vi "DataProcessScaleAdjust.vi"(8 "error in (no error)":errorcluster, 10 "Graph":dbl[](array[numeric]), 11 "Graph":refnum<vi>) -> (0 "error out":errorcluster, 3 "reference out":refnum<vi>)   [LabVIEW 2013, in "main.lvlib"]
uses:
  main.lvlib
  <vilib>/Utility/miscctls.llb/LVRangeTypeDef.ctl
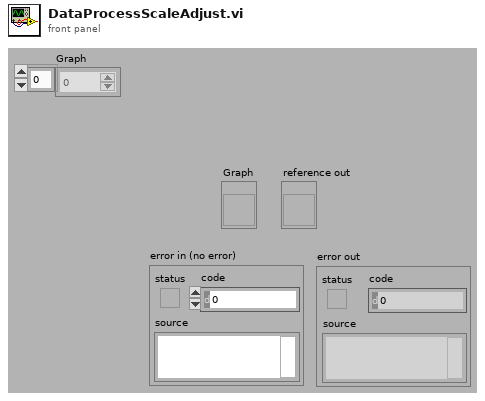
[diagram p1: front panel]
types:
  T1 = typedef "LVRangeTypeDef.ctl" = cluster{"Minimum":dbl, "Maximum":dbl, "Increment":dbl, "Minor Increment":dbl, "Start":dbl}
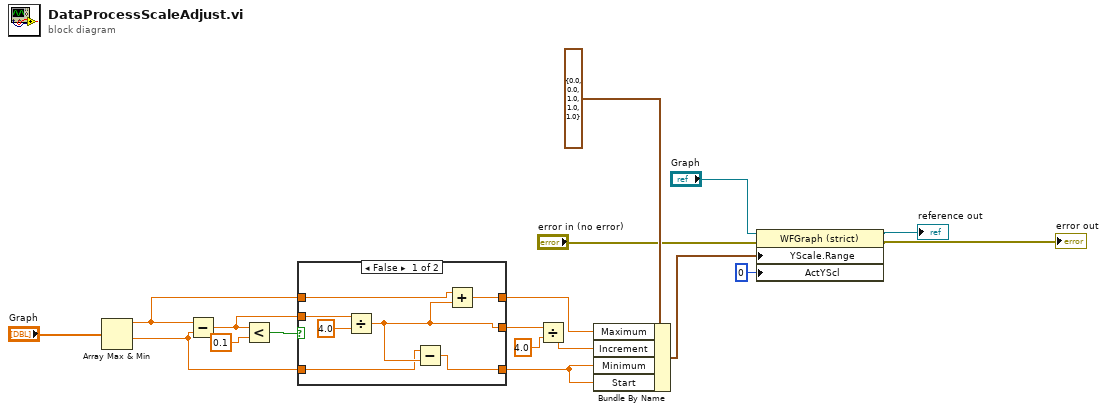
[diagram p0: block diagram]
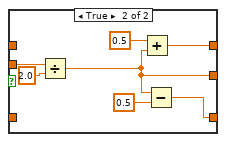
[diagram p2: hidden frame]
diagram:
  n1 = Array Max & Min(array="Graph") -> (max value=w4:dbl, min value=w5:dbl)  [unwired: 2 out]
  n2 = Subtract(x=w4, y=w5) -> (x-y=w9:dbl)
  n3 = Less?(x=w9, y=0.1) -> (x < y?=w10:bool)
  n4 = case shown="False" w10 {
    tunnel: w9 -> [w25 w31]
    tunnel: [w21 w27] -> w8
    tunnel: w5 -> [w20 _]
    tunnel: [w19 w28] -> w7
    tunnel: [w23 w26] -> w6
    tunnel: w4 -> [w22 _]
    frame False {
      n5 = Divide(x=w25, y=4.0) -> (x/y=w21:dbl)
      n6 = Subtract(x=w20, y=w21) -> (x-y=w19:dbl)
      n7 = Add(x=w22, y=w21) -> (x+y=w23:dbl)
    }
    frame True {
      n8 = Divide(x=w31, y=2.0) -> (x/y=w27:dbl)
      n9 = Add(x=0.5, y=w27) -> (x+y=w26:dbl)
      n10 = Subtract(x=w27, y=0.5) -> (x-y=w28:dbl)
    }
  }
  n11 = Divide(x=w8, y=4.0) -> (x/y=w15:dbl)
  n12 = Bundle By Name(cluster=T1 {"Minimum"=0.0, "Maximum"=0.0, "Increment"=1.0, "Minor Increment"=1.0, "Start"=1.0} ("Y Scale.Range"), "Maximum"=w6, "Increment"=w15, "Minimum"=w7, "Start"=w7) -> (w17:T1)
  n13 = property class="WFGraph (strict)"(reference="Graph", error in="error in (no error)", "YScale.Range"=w17, "ActYScl"=0 ("Active Y Scale")) -> (reference out=→"reference out":refnum<vi>, error out=→"error out":errorcluster)
